vi "link - optimal2.vi"(8 "dc44":dbl[](array[numeric]), 9 "dc11":dbl[](array[numeric]), 10 "freqs 2":dbl[](array[numeric]), 11 "freqs 1":dbl[](array[numeric])) -> (0 "beta opt":dbl, 1 "alpha opt":dbl)   [LabVIEW 2014]
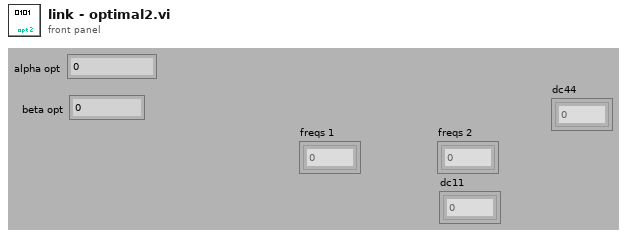
[diagram p1: front panel]
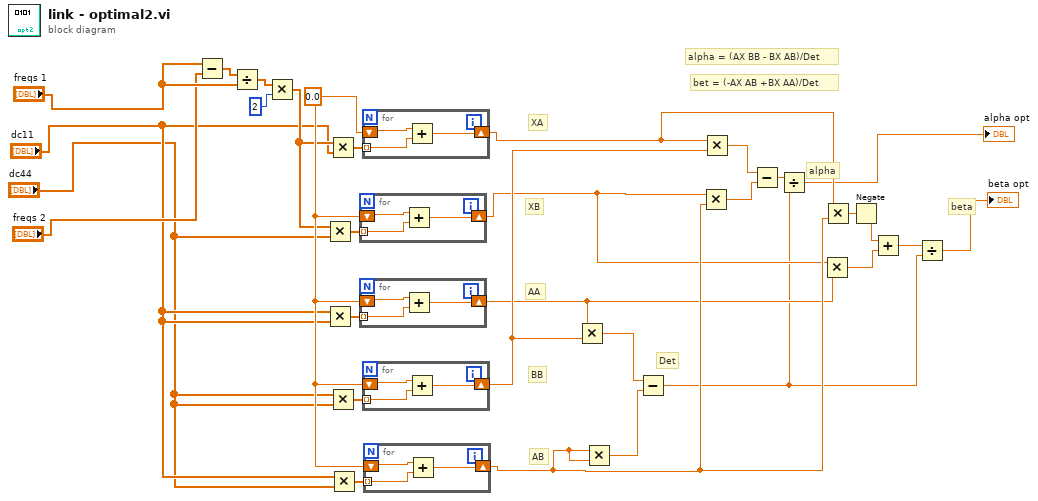
[diagram p0: block diagram]
diagram:
  w23 = 0.0
  # "beta"
  # "alpha"
  # "bet = (-AX AB +BX AA)/Det"
  # "alpha = (AX BB - BX AB)/Det"
  # "Det"
  # "AB"
  # "BB"
  # "AA"
  # "XB"
  # "XA"
  n1 = Subtract(x="freqs 1", y="freqs 2") -> (x-y=w31:dbl[])
  n2 = Divide(x=w31, y="freqs 1") -> (x/y=w30:dbl[])
  n3 = Multiply(x=w30, y=2) -> (x*y=w22:dbl[])
  n4 = Multiply(x=w22, y="dc44") -> (x*y=w27:dbl[])
  n5 = Multiply(x="dc11", y="dc11") -> (x*y=w26:dbl[])
  n6 = Multiply(x=w22, y="dc11") -> (x*y=w28:dbl[])
  n7 = Multiply(x="dc44", y="dc44") -> (x*y=w25:dbl[])
  n8 = Multiply(x="dc11", y="dc44") -> (x*y=w24:dbl[])
  n9 = for {
    shift-right: [w33] -> w9
    shift-left: w23 -> [w34]
    tunnel: w27 -> [w32] mode=indexing
    n10 = Add(x=w34, y=w32) -> (x+y=w33:dbl)
  }
  n11 = for {
    shift-right: [w36] -> w8
    shift-left: w23 -> [w37]
    tunnel: w26 -> [w35] mode=indexing
    n12 = Add(x=w37, y=w35) -> (x+y=w36:dbl)
  }
  n13 = for {
    shift-right: [w39] -> w13
    shift-left: w23 -> [w40]
    tunnel: w28 -> [w38] mode=indexing
    n14 = Add(x=w40, y=w38) -> (x+y=w39:dbl)
  }
  n15 = for {
    shift-right: [w42] -> w17
    shift-left: w23 -> [w43]
    tunnel: w25 -> [w41] mode=indexing
    n16 = Add(x=w43, y=w41) -> (x+y=w42:dbl)
  }
  n17 = for {
    shift-right: [w45] -> w12
    shift-left: w23 -> [w46]
    tunnel: w24 -> [w44] mode=indexing
    n18 = Add(x=w46, y=w44) -> (x+y=w45:dbl)
  }
  n19 = Multiply(x=w8, y=w17) -> (x*y=w20:dbl)
  n20 = Multiply(x=w12, y=w12) -> (x*y=w21:dbl)
  n21 = Subtract(x=w20, y=w21) -> (x-y=w7:dbl)
  n22 = Multiply(x=w9, y=w12) -> (x*y=w19:dbl)
  n23 = Multiply(x=w13, y=w17) -> (x*y=w18:dbl)
  n24 = Subtract(x=w18, y=w19) -> (x-y=w16:dbl)
  n25 = Divide(x=w16, y=w7) -> (x/y=→"alpha opt":dbl)
  n26 = Multiply(x=w9, y=w8) -> (x*y=w15:dbl)
  n27 = Multiply(x=w13, y=w12) -> (x*y=w11:dbl)
  n28 = Negate(x=w11) -> (-x=w10:dbl)
  n29 = Add(x=w10, y=w15) -> (x+y=w14:dbl)
  n30 = Divide(x=w14, y=w7) -> (x/y=→"beta opt":dbl)
